vi "Joystick Drive.vi"   [LabVIEW 2013]
types:
  T1 = cluster{"Joystick 1 X axis":dbl, "Joystick 1 Y axis":dbl, "Triggers":dbl, "Joystick 2 X axis":dbl, "Joystick 2 Y axis":dbl, "axis 6":dbl}
  T2 = typedef "WPI_JoystickButtonState.ctl" = cluster{"Button 1":bool, "Button 2":bool, "Button 3":bool, "Button 4":bool, "Button 5":bool, "Button 6":bool, "Button 7":bool, "Button 8":bool, "Button 9":bool, "Button 10":bool, "Button 11":bool, "Button 12":bool}
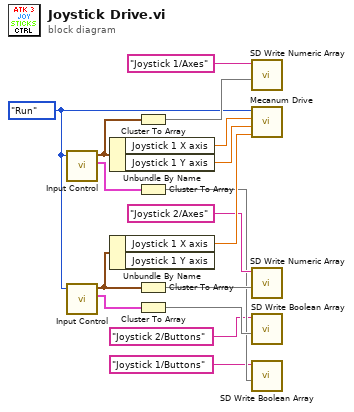
[diagram p0: block diagram]
diagram:
  w3 = enum16{"Open", "Run", "End"}."Run" ("State")
  n1 = call "Input Control.vi"("State"=w3) -> ("Axes"=w4:T1, "Buttons"=w5:T2)  [unwired: 3 in, 1 out]
  n2 = call "Input Control.vi"("State"=w3) -> ("Axes"=w1:T1, "Buttons"=w2:T2)  [unwired: 3 in, 1 out]
  n3 = Unbundle By Name(w4) -> ("Joystick 1 X axis"=w16:dbl, "Joystick 1 Y axis"=w15:dbl)
  n4 = Unbundle By Name(w1) -> ("Joystick 1 X axis"=w14:dbl)  [unwired: 1 out]
  n5 = Cluster To Array(cluster=w4) -> (array=w11:dbl[])
  n6 = Cluster To Array(cluster=w5) -> (array=w8:bool[])
  n7 = Cluster To Array(cluster=w1) -> (array=w13:dbl[])
  n8 = Cluster To Array(cluster=w2) -> (array=w9:bool[])
  n9 = call <vilib>:"SD Write Numeric Array.vi"("Numeric Array"=w11, "Name"="Joystick 1/Axes") -> ()  [unwired: 8 in, 2 out]
  n10 = call "Mecanum Drive.vi"("Turning"=w14, "F/R"=w15, "Strafing"=w16, "State Control"=w3) -> ()
  n11 = call <vilib>:"SD Write Numeric Array.vi"("Numeric Array"=w13, "Name"="Joystick 2/Axes") -> ()  [unwired: 8 in, 2 out]
  n12 = call <vilib>:"SD Write Boolean Array.vi"("Boolean Array"=w9, "Name"="Joystick 2/Buttons") -> ()  [unwired: 8 in, 2 out]
  n13 = call <vilib>:"SD Write Boolean Array.vi"("Boolean Array"=w8, "Name"="Joystick 1/Buttons") -> ()  [unwired: 8 in, 2 out]
